vi "Armstrong_Number_Check.vi"() -> ()   [LabVIEW 2026]
panel:
  out "Armstrong Check Result":bool
  out "Calculated Armstrong Value":dbl
  in  "Number Under Test":i32
  # "Title -"
  # "Armstrong Number Check"
  # "Demonstrates While Loop-based digit extraction and arithmetic operations \nto determine whether a number is an Armstrong number."
  # "Description -"
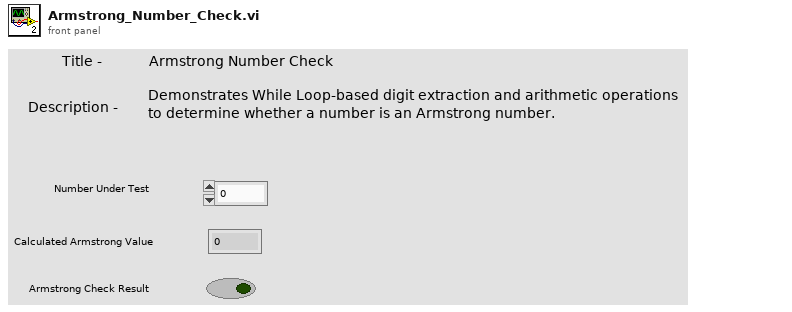
[diagram p1: front panel]
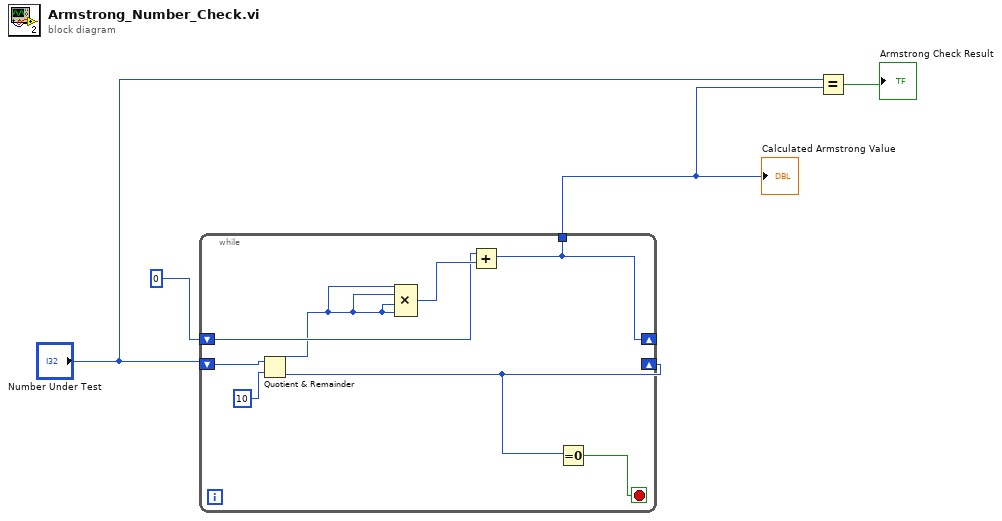
[diagram p0: block diagram]
diagram:
  n1 = while {
    shift-right: [w10] -> _
    shift-left: "Number Under Test" -> [w12]
    shift-right: [w7] -> _
    shift-left: 0 -> [w6]
    tunnel: [w7] -> w3
    stop <- w9 stop-if-true
    n2 = Quotient & Remainder(x=w12, y=10) -> (x-y*floor(x/y)=w5:i32, floor(x/y)=w10:i32)
    n3 = Compound Arithmetic op=MULTIPLY(w5, w5, w5, w5) -> (w8:i32)
    n4 = Add(x=w6, y=w8) -> (x+y=w7:i32)
    n5 = Equal To 0?(x=w10) -> (x = 0?=w9:bool)
  }
  "Calculated Armstrong Value" <- w3
  n6 = Equal?(x="Number Under Test", y=w3) -> (x = y?=→"Armstrong Check Result":bool)
